vi "Initialize shutter.vi"(8 "error in":errorcluster, 9 "Main cluster in":T1, 11 "Device":tag="APD_Count") -> (0 "error out":errorcluster, 1 "Main cluster out":T1)   [LabVIEW 2010]
uses:
  Main_cluster.ctl
  <vilib>/DAQmx/create/channels.llb/DAQmx Create Channel (DO-Digital Output).vi
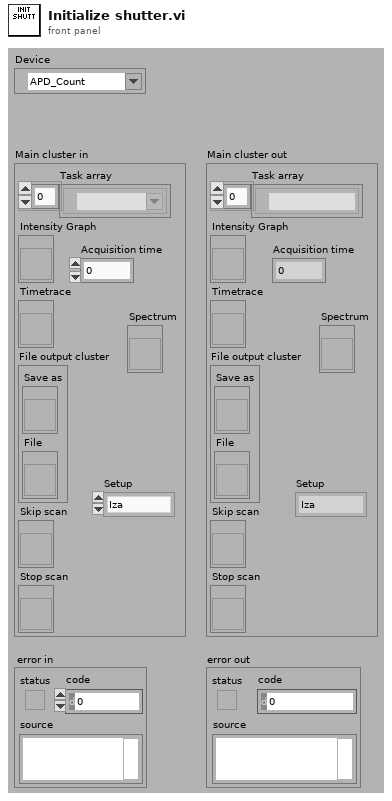
[diagram p1: front panel]
types:
  T1 = typedef "Main_cluster.ctl" = cluster{"Task array":refnum<k21>[], "Intensity Graph":refnum<vi>, "Timetrace":refnum<vi>, "File output cluster":cluster{"Save as":refnum<vi>, "File":refnum<vi>}, "Skip scan":refnum<vi>, "Stop scan":refnum<vi>, "Acquisition time":dbl, "Setup":enum16{"Iza", "Lukasz"}, "Spectrum":refnum<vi>}
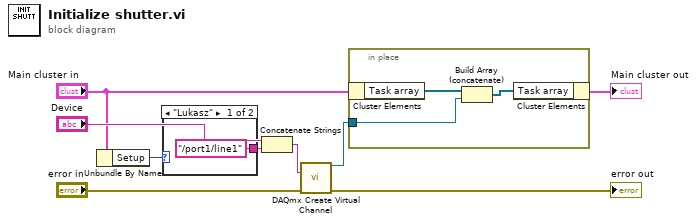
[diagram p0: block diagram]
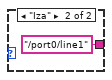
[diagram p2: hidden frame]
diagram:
  n1 = Unbundle By Name("Main cluster in") -> ("Setup"=w2:enum16{"Iza", "Lukasz"})
  n2 = case shown="\"Lukasz\"" w2 {
    tunnel: ["/port1/line1" ("string") "/port0/line1" ("string")] -> w8
    frame "Lukasz" {
    }
    frame "Iza" {
    }
  }
  n3 = Concatenate Strings("Device", w8) -> (w5:string)
  n4 = call-poly <vilib>:"DAQmx Create Virtual Channel.vi"("lines"=w5, "error in"="error in") -> ("task out"=w3:refnum<k21>, "error out"=→"error out":errorcluster)  [unwired: 12 in]
  n5 = in-place {
    in-place-border: w3 -> [w12]
    n6 = in-place-cluster #1("Main cluster in") -> ("Task array"=w14:refnum<k21>[])
    n7 = Build Array (concatenate)(w14, w12) -> (w13:refnum<k21>[])
    n8 = in-place-cluster #1("Task array"=w13) -> (→"Main cluster out":T1)
  }
